vi "SolarPVLab.vi"(0 "SHDocVw.IWebBrowser2":refnum<k7>(container), 1 "location :":string, 2 "Go":bool) -> ()   [LabVIEW 2011]
doc: "To use this browser, you can type in a URL in the location field and then click on the Go button. You can also use the Back, Forward, Reload and Search buttons. This VI also has a runtime menu which is included in the library. When you run the VI, you will have File Menu and a History Menu. The file menu contains the same functionality that the buttons can do and the History menu contains a History of all the pages that you have visited in a given session.\n\nThe Invoke Node and Property Node functions are used to control the operation of the web browser. For more information on the Microsoft Web Browser Control, see Microsoft's web site (try http://support.microsoft.com/support/kb/articles/q165/2/12.asp)."
uses:
  2009 final/Solar Pv project Folder/SolarPVLab Folder/Voltage Array1.vi
panel:
  out "Current 150":dbl[](array[numeric])
  out "Voltage 150":dbl[](array[numeric])
  out "Current 130":dbl[](array[numeric])
  out "Voltage 130":dbl[](array[numeric])
  out "Current 100":dbl[](array[numeric])
  out "Voltage 100":dbl[](array[numeric])
  out "Current 60":dbl[](array[numeric])
  out "Voltage 60":dbl[](array[numeric])
  in  "stop":bool
  out "Video Feed":T1(plugin-control)
  in  "Tab Control":T2(tab)
  in  "Search":bool
  in  "Reload":bool
  in  "Back":bool
  in  "Forward":bool
  in  "Irradiation":T3(ring)
  in  "Resistance":T4(ring)
  in  "Angle of Incidence":T5(ring)
  out "Current Values Plotted":T6
  in  "Plot Current Values":T7
  in  "Plot Voltage Values":T8
  out "Voltage Values Plotted":T9
  in  "Tab Control 2":T10(tab)
  out "IV characeristics":cluster{"Y":dbl[], "Y":dbl[]}[](graph)
  out "Power vs Voltage":cluster{"Y":dbl[], "Y":dbl[]}[](graph)
  out "Current vs Incidence":cluster{"Y":dbl[], "Y":dbl[]}[](graph)
  out "Voltage vs Incidence":cluster{"Y":dbl[], "Y":dbl[]}[](graph)
  out "Irradiation Graph":cluster{dbl[], dbl[]}[](graph)
  out "Power varying with Irradiation Graph":cluster{dbl[], dbl[]}[](graph)
  out "Passing Array":string[](array[string])=["http://espn.go.com/", "http://www.natinst.com/"]
  # "WELCOME TO THE SOLAR PHOTOVOLTAIC LABORATORY\n\n\n\n\nTHIS SOLAR PHOTOVOLTAIC ILAB INVESTIGATES THE FOLLOWING \n                  CHARACTERISTICS OF A SOLAR PANEL:\n\n~CURRENT - VOLTAGE (IV) CHARACTERISITICS\n~VARIATION OF IV CHARACTERISITCS WITH IRRADIATION\n~VARIATION OF CURRENT AND VOLTAGE WITH ANGLE OF INCIDENCE\n\n\n\n\n\n\n© 2014 iLABS@MAK"
  # "* Select VI Info... from the Windows menu to find out how to use this example. *"
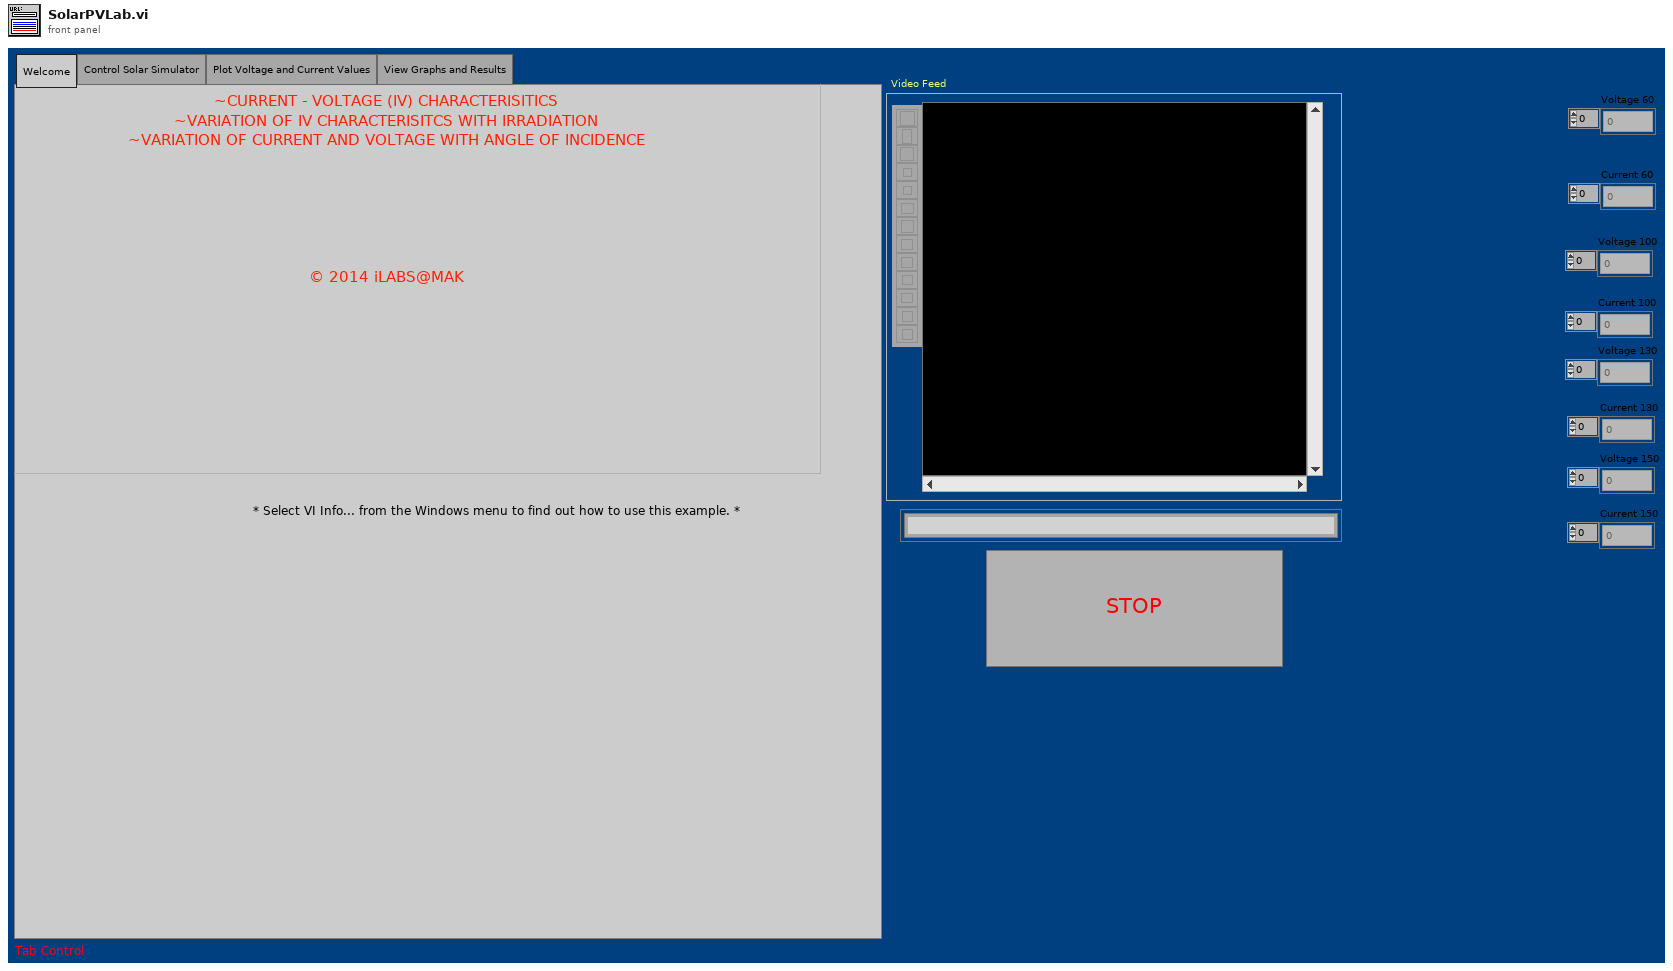
[diagram p1: front panel]
types:
  T1 = typedef "IMAQ Image.ctl" = refnum<image>
  T2 = enum32{"Welcome", "Control Solar Simulator", "Plot Voltage and Current Values", "View Graphs and Results"}
  T3 = enum16{"Choose Irradiation", "60", "100", "130", "150"}
  T4 = enum16{"Choose Resistance", "2.2 ohms", "4.7 ohms", "6.8 ohms", "8.2 ohms", "10 ohms", "12 ohms", "Shortciruit"}
  T5 = enum16{"0", "20", "40", "60", "80", "100", "120", "140", "160", "180"}
  T6 = cluster{"Short circuit\n current":dbl, "Value 1":dbl, "Value 2":dbl, "Value 3":dbl, "Value 4":dbl, "Value 5":dbl, "Value 6":dbl}
  T7 = cluster{"Plot Short \nCircuit current":bool, "Plot Value 2":bool, "Plot Value 3":bool, "Plot Value 4":bool, "Plot Value 5":bool, "Plot Value 6":bool, "Plot Value 7":bool}
  T8 = cluster{"Plot Value 1":bool, "Plot Value 2":bool, "Plot Value 3":bool, "Plot Value 4":bool, "Plot Value 5":bool, "Plot Value 6":bool, "Plot Open Circuit Voltage":bool}
  T9 = cluster{"Value 1":dbl, "Value 2":dbl, "Value 3":dbl, "Value 4":dbl, "Value 5":dbl, "Value 6":dbl, "Open circuit \n    Voltage":dbl}
  T10 = enum32{"IV Characteristics", "Power vs Voltage Graph", "Variation with Angle of Incidence", "IV-Variation with Irradiation", "Power-Irradiation Graph"}
  T11 = cluster{dynamicdata, dynamicdata, dynamicdata, dynamicdata, dynamicdata, dynamicdata, dynamicdata}
  T12 = cluster{"Voltage 150":dbl[], "Current 150":dbl[]}
  T13 = cluster{"Voltage 130":dbl[], "Current 130":dbl[]}
  T14 = cluster{"Voltage 100":dbl[], "Current 100":dbl[]}
  T15 = cluster{"Voltage 150":dbl[], "Current 150":dbl[]}[]
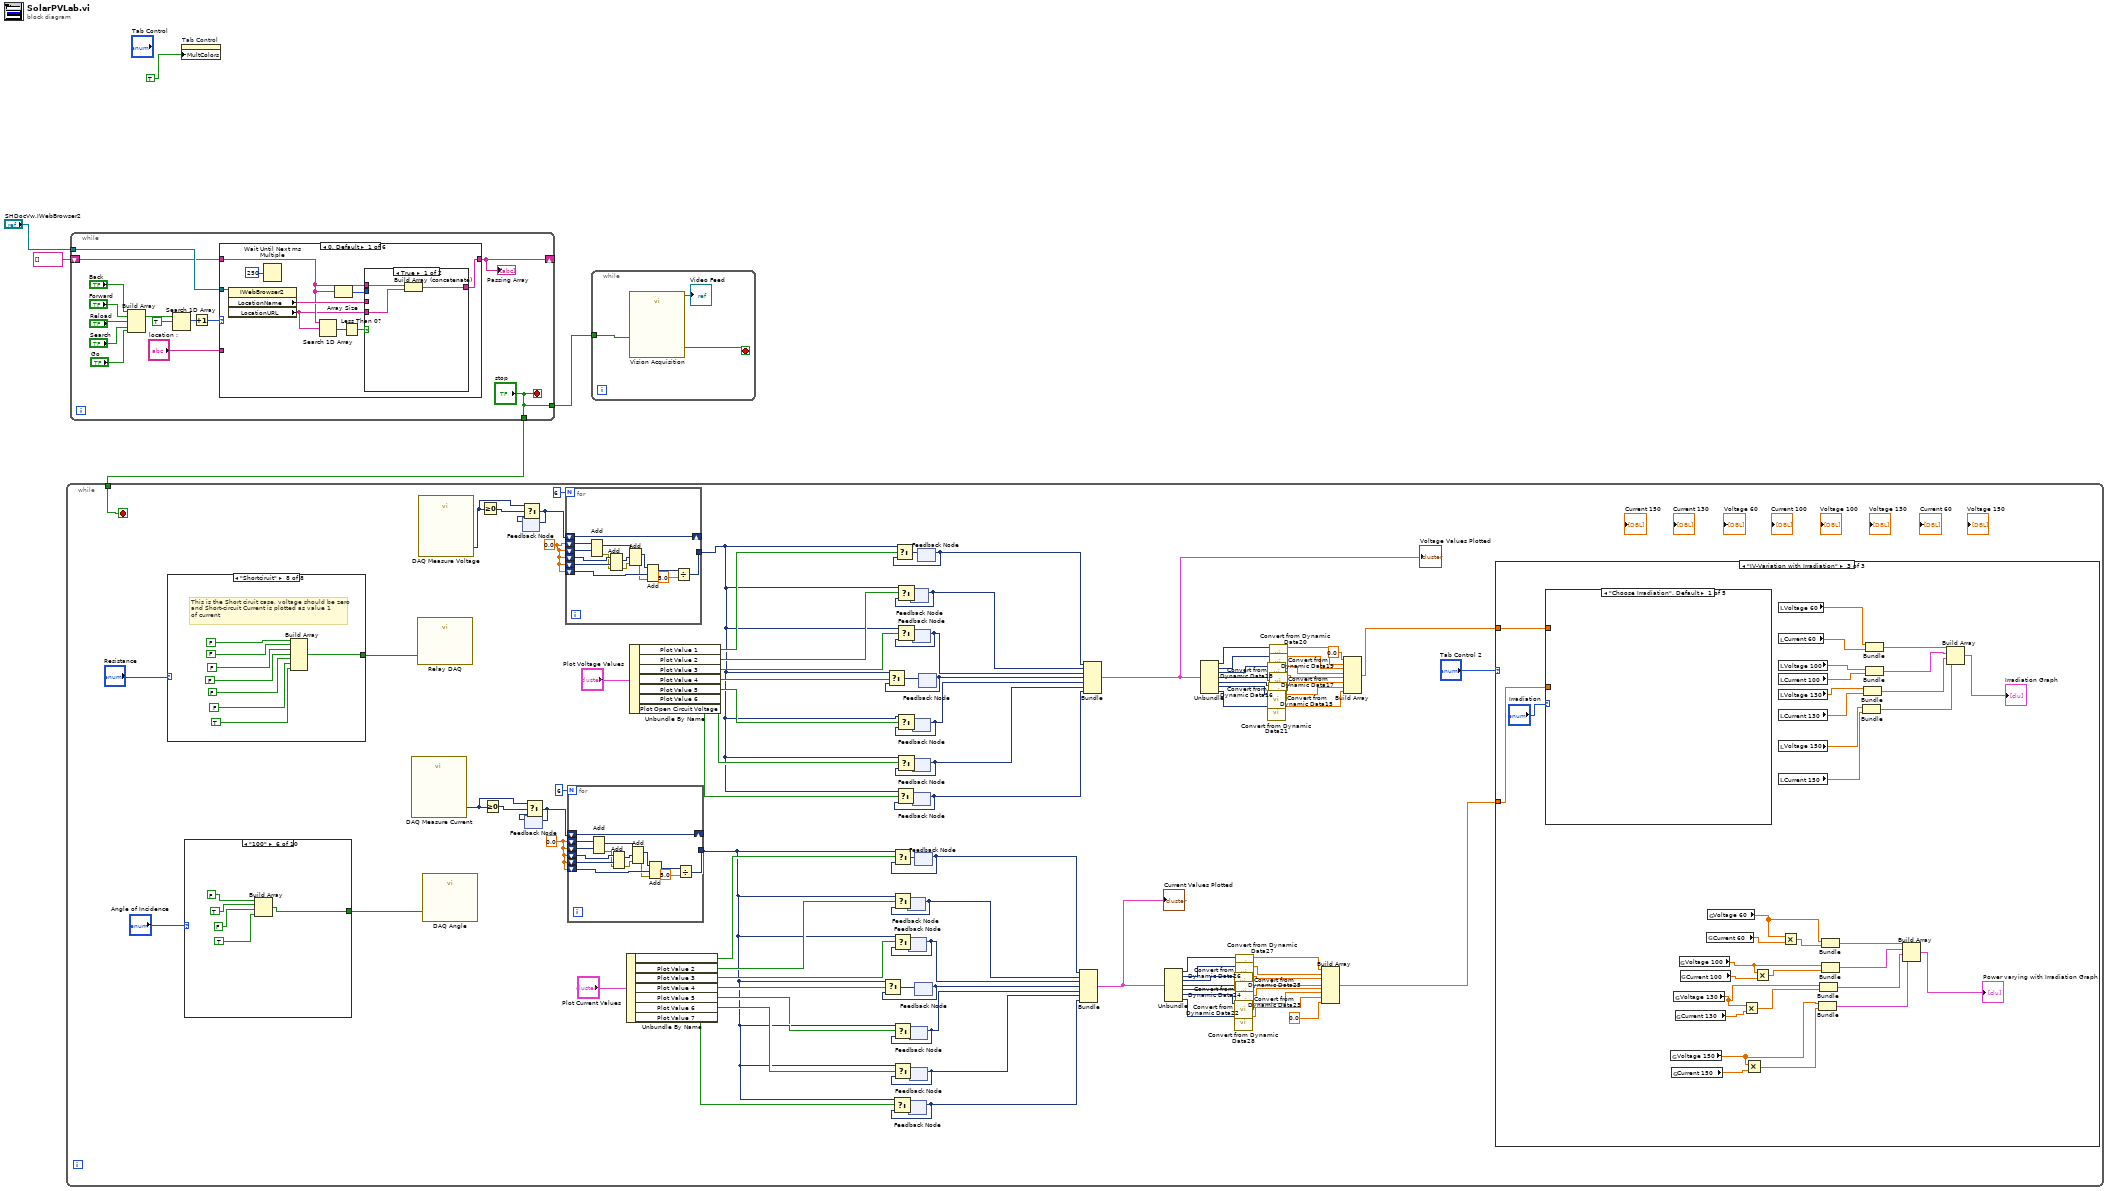
[diagram p0: block diagram]
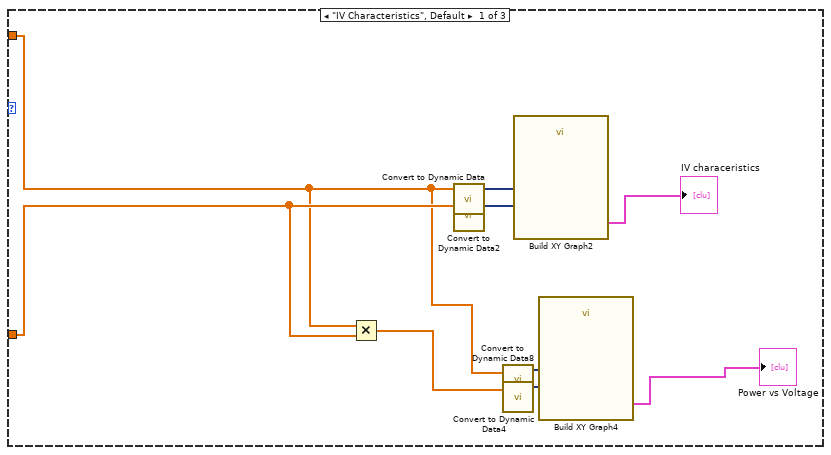
[diagram p2: hidden frame]
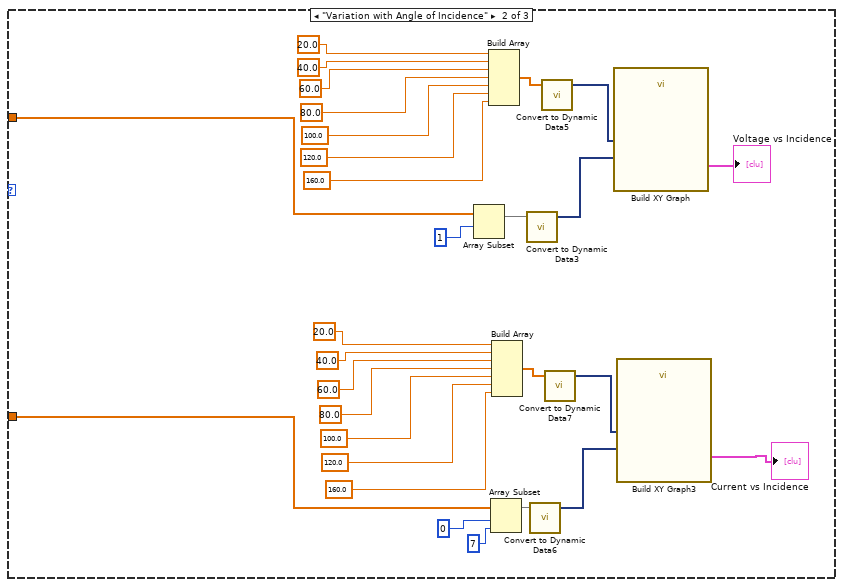
[diagram p3: hidden frame]
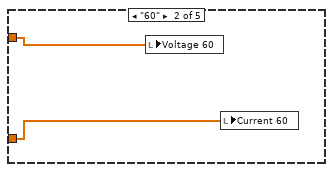
[diagram p4: hidden frame]
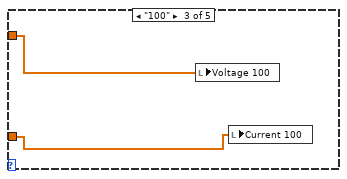
[diagram p5: hidden frame]
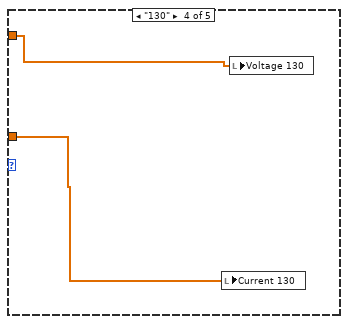
[diagram p6: hidden frame]
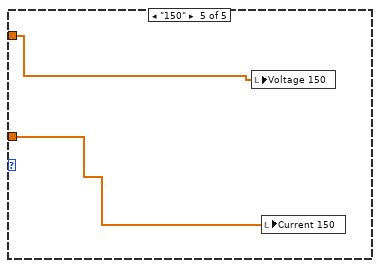
[diagram p7: hidden frame]
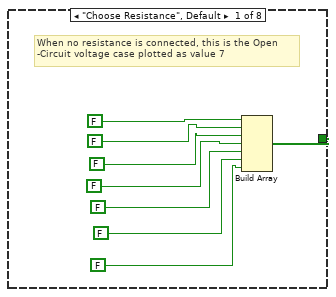
[diagram p8: hidden frame]
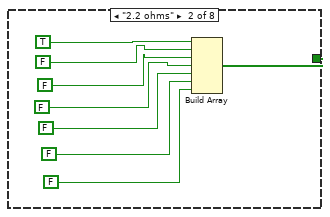
[diagram p9: hidden frame]
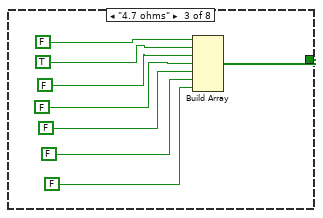
[diagram p10: hidden frame]
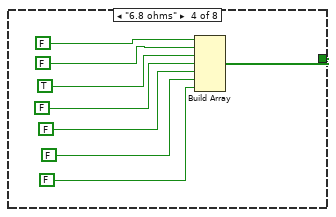
[diagram p11: hidden frame]
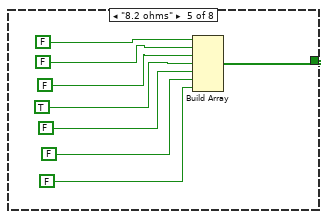
[diagram p12: hidden frame]
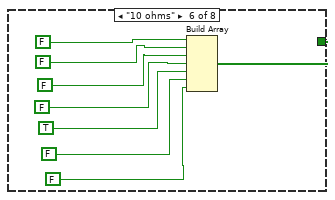
[diagram p13: hidden frame]
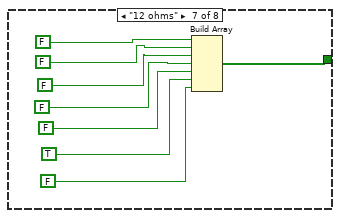
[diagram p14: hidden frame]
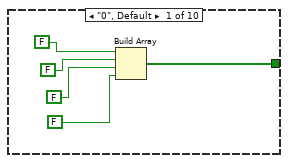
[diagram p15: hidden frame]
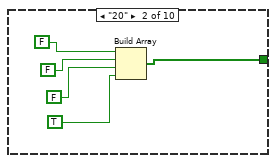
[diagram p16: hidden frame]
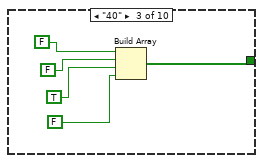
[diagram p17: hidden frame]
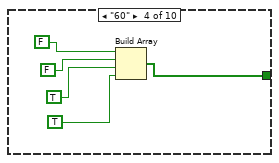
[diagram p18: hidden frame]
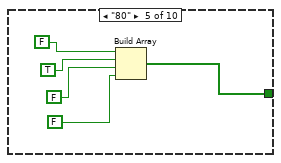
[diagram p19: hidden frame]
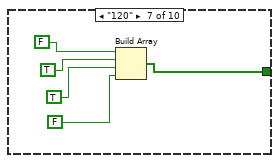
[diagram p20: hidden frame]
diagram:
  n1 = while {
    shift-left: string[] [] -> [w9]
    shift-right: [w8] -> _
    tunnel: "SHDocVw.IWebBrowser2" -> [w10]
    tunnel: ["stop"] -> w2
    tunnel: ["stop"] -> w1
    stop <- "stop" stop-if-true
    n2 = Build Array("Back", "Forward", "Reload", "Search", "Go") -> (w14:bool[])
    n3 = Search 1D Array(1D array=w14, element=TRUE) -> (index of element=w12:i32)  [unwired: 1 in]
    n4 = Increment(x=w12) -> (x+1=w11:i32)
    n5 = case shown="0, Default" w11 {
      tunnel: w10 -> [w20 w34 w36 w37 w39 w43]
      tunnel: "location :" -> [_ _ _ _ _ w42]
      tunnel: w9 -> [w24 w33 w35 w38 w40 w41]
      tunnel: [w23 w33 w35 w38 w40 w41] -> w8
      frame 0, Default {
        n6 = property class="IWebBrowser2"(reference=w20) -> ("LocationName"=w28:string, "LocationURL"=w21:string)  [unwired: 1 in, 2 out]
        n7 = Wait Until Next ms Multiple(millisecond multiple=u32 250) -> ()  [unwired: 1 out]
        n8 = Search 1D Array(1D array=w24, element=w21) -> (index of element=w27:i32)  [unwired: 1 in]
        n9 = Array Size(array=w24) -> (size(s)=w25:i32)
        n10 = Less Than 0?(x=w27) -> (x < 0?=w26:bool)
        n11 = case shown="True" w26 {
          tunnel: w28 -> [_ _]
          tunnel: w21 -> [w29 _]
          tunnel: w25 -> [_ _]
          tunnel: w24 -> [w31 w32]
          tunnel: [w30 w32] -> w23
          frame True {
            n12 = Build Array (concatenate)(w31, w29) -> (w30:string[])
          }
          frame False {
          }
        }
      }
      frame 1 {
        n13 = invoke class="IWebBrowser2" method="GoBack"(reference=w34) -> ()  [unwired: 2 in, 3 out]
      }
      frame 2 {
        n14 = invoke class="IWebBrowser2" method="GoForward"(reference=w36) -> ()  [unwired: 2 in, 3 out]
      }
      frame 3 {
        n15 = invoke class="IWebBrowser2" method="Refresh"(reference=w37) -> ()  [unwired: 2 in, 3 out]
      }
      frame 4 {
        n16 = invoke class="IWebBrowser2" method="GoSearch"(reference=w39) -> ()  [unwired: 2 in, 3 out]
      }
      frame 5 {
        n17 = invoke class="IWebBrowser2" method="Navigate"(reference=w43, "URL"=w42) -> ()  [unwired: 6 in, 8 out]
      }
    }
    "Passing Array" <- w8
  }
  n18 = while {
    tunnel: w2 -> [w44]
    stop <- w44 stop-if-true
    w45 = 0.0
    w46 = 0.0
    n19 = case shown="\"Shortciruit\"" "Resistance" {
      tunnel: [w252 w260 w268 w276 w284 w292 w300 w307] -> w139
      frame "Choose Resistance", Default {
        # "When no resistance is connected, this is the Open\n-Circuit voltage case plotted as value 7"
        n20 = Build Array(FALSE, FALSE, FALSE, FALSE, FALSE, FALSE, FALSE) -> (w252:bool[])
      }
      frame "2.2 ohms" {
        n21 = Build Array(TRUE, FALSE, FALSE, FALSE, FALSE, FALSE, FALSE) -> (w260:bool[])
      }
      frame "4.7 ohms" {
        n22 = Build Array(FALSE, TRUE, FALSE, FALSE, FALSE, FALSE, FALSE) -> (w268:bool[])
      }
      frame "6.8 ohms" {
        n23 = Build Array(FALSE, FALSE, TRUE, FALSE, FALSE, FALSE, FALSE) -> (w276:bool[])
      }
      frame "8.2 ohms" {
        n24 = Build Array(FALSE, FALSE, FALSE, TRUE, FALSE, FALSE, FALSE) -> (w284:bool[])
      }
      frame "10 ohms" {
        n25 = Build Array(FALSE, FALSE, FALSE, FALSE, TRUE, FALSE, FALSE) -> (w292:bool[])
      }
      frame "12 ohms" {
        n26 = Build Array(FALSE, FALSE, FALSE, FALSE, FALSE, TRUE, FALSE) -> (w300:bool[])
      }
      frame "Shortciruit" {
        # "This is the Short ciruit case, voltage should be zero \nand Short-circuit Current is plotted as value 1 \nof current"
        n27 = Build Array(FALSE, FALSE, FALSE, FALSE, FALSE, FALSE, TRUE) -> (w307:bool[])
      }
    }
    n28 = case shown="\"100\"" "Angle of Incidence" {
      tunnel: [w315 w320 w325 w330 w335 w340 w345 w350 w355 w360] -> w140
      frame "0", Default {
        n29 = Build Array(FALSE, FALSE, FALSE, FALSE) -> (w315:bool[])
      }
      frame "20" {
        n30 = Build Array(FALSE, FALSE, FALSE, TRUE) -> (w320:bool[])
      }
      frame "40" {
        n31 = Build Array(FALSE, FALSE, TRUE, FALSE) -> (w325:bool[])
      }
      frame "60" {
        n32 = Build Array(FALSE, FALSE, TRUE, TRUE) -> (w330:bool[])
      }
      frame "80" {
        n33 = Build Array(FALSE, TRUE, FALSE, FALSE) -> (w335:bool[])
      }
      frame "100" {
        n34 = Build Array(FALSE, TRUE, FALSE, TRUE) -> (w340:bool[])
      }
      frame "120" {
        n35 = Build Array(FALSE, TRUE, TRUE, FALSE) -> (w345:bool[])
      }
      frame "140" {
        n36 = Build Array(FALSE, TRUE, TRUE, TRUE) -> (w350:bool[])
      }
      frame "160" {
        n37 = Build Array(TRUE, FALSE, FALSE, FALSE) -> (w355:bool[])
      }
      frame "180" {
        n38 = Build Array(TRUE, FALSE, FALSE, TRUE) -> (w360:bool[])
      }
    }
    n39 = call "DAQ Measure Current"() -> ("data"=w57:dynamicdata)  [unwired: 17 in, 2 out]
    n40 = call "Relay DAQ"("data"=w139) -> ()  [unwired: 17 in, 2 out]
    n41 = call "DAQ Measure Voltage"() -> ("data"=w50:dynamicdata)  [unwired: 17 in, 2 out]
    n42 = call "DAQ Angle"("data"=w140) -> ()  [unwired: 17 in, 2 out]
    n43 = Greater Or Equal To 0?(x=w50) -> (x >= 0?=w53:dynamicdata)
    n44 = Greater Or Equal To 0?(x=w57) -> (x >= 0?=w58:dynamicdata)
    n45 = feedback #1() -> (w52:dynamicdata)  [unwired: 1 in]
    n46 = Select(t=w50, s=w53, f=w52) -> (s? t:f=w51:dynamicdata)
    n47 = feedback-in #1(w51) -> ()
    n48 = feedback #2() -> (w56:dynamicdata)  [unwired: 1 in]
    n49 = Select(t=w57, s=w58, f=w56) -> (s? t:f=w55:dynamicdata)
    n50 = feedback-in #2(w55) -> ()
    n51 = for {
      N: 6 -> [_]
      shift-right: [w156] -> _
      shift-left: w51 -> [w156]
      shift-left: w45 -> [w155]
      shift-left: w45 -> [w154]
      shift-left: w45 -> [w153]
      shift-left: w45 -> [w152]
      shift-left: w45 -> [w148]
      tunnel: [w145] -> w49
      n52 = Add(1:w154, 2:w155) -> (0:w151:dynamicdata, 3:w144:errorcluster)  [unwired: 1 in]
      n53 = Add(1:w152, 2:w153, 4:w144) -> (0:w150:dynamicdata, 3:w143:errorcluster)
      n54 = Add(1:w150, 2:w151, 4:w143) -> (0:w149:dynamicdata, 3:w142:errorcluster)
      n55 = Add(1:w148, 2:w149, 4:w142) -> (0:w147:dynamicdata)  [unwired: 1 out]
      n56 = Divide(x=w147, y=5.0) -> (x/y=w145:dynamicdata)
    }
    n57 = for {
      N: 6 -> [_]
      shift-right: [w171] -> _
      shift-left: w55 -> [w171]
      shift-left: w46 -> [w170]
      shift-left: w46 -> [w169]
      shift-left: w46 -> [w168]
      shift-left: w46 -> [w167]
      shift-left: w46 -> [w163]
      tunnel: [w160] -> w54
      n58 = Add(1:w169, 2:w170) -> (0:w166:dynamicdata, 3:w159:errorcluster)  [unwired: 1 in]
      n59 = Add(1:w167, 2:w168, 4:w159) -> (0:w165:dynamicdata, 3:w158:errorcluster)
      n60 = Add(1:w165, 2:w166, 4:w158) -> (0:w164:dynamicdata, 3:w157:errorcluster)
      n61 = Add(1:w163, 2:w164, 4:w157) -> (0:w162:dynamicdata)  [unwired: 1 out]
      n62 = Divide(x=w162, y=5.0) -> (x/y=w160:dynamicdata)
    }
    n63 = Unbundle By Name("Plot Current Values") -> ("Plot Short \nCircuit current"=w103:bool, "Plot Value 2"=w102:bool, "Plot Value 3"=w101:bool, "Plot Value 4"=w100:bool, "Plot Value 5"=w99:bool, "Plot Value 6"=w59:bool, "Plot Value 7"=w79:bool)
    n64 = Unbundle By Name("Plot Voltage Values") -> ("Plot Value 1"=w68:bool, "Plot Value 2"=w67:bool, "Plot Value 3"=w66:bool, "Plot Value 4"=w65:bool, "Plot Value 5"=w64:bool, "Plot Value 6"=w63:bool, "Plot Open Circuit Voltage"=w62:bool)
    n65 = feedback #3() -> (w98:dynamicdata)  [unwired: 1 in]
    n66 = Select(t=w54, s=w102, f=w98) -> (s? t:f=w108:dynamicdata)
    n67 = feedback-in #3(w108) -> ()
    n68 = feedback #4() -> (w97:dynamicdata)  [unwired: 1 in]
    n69 = Select(t=w54, s=w101, f=w97) -> (s? t:f=w107:dynamicdata)
    n70 = feedback-in #4(w107) -> ()
    n71 = feedback #5() -> (w78:dynamicdata)  [unwired: 1 in]
    n72 = Select(t=w54, s=w79, f=w78) -> (s? t:f=w80:dynamicdata)
    n73 = feedback-in #5(w80) -> ()
    n74 = feedback #6() -> (w95:dynamicdata)  [unwired: 1 in]
    n75 = Select(t=w54, s=w99, f=w95) -> (s? t:f=w105:dynamicdata)
    n76 = feedback-in #6(w105) -> ()
    n77 = feedback #7() -> (w94:dynamicdata)  [unwired: 1 in]
    n78 = Select(t=w54, s=w59, f=w94) -> (s? t:f=w104:dynamicdata)
    n79 = feedback-in #7(w104) -> ()
    n80 = feedback #8() -> (w129:dynamicdata)  [unwired: 1 in]
    n81 = Select(t=w49, s=w67, f=w129) -> (s? t:f=w134:dynamicdata)
    n82 = feedback-in #8(w134) -> ()
    n83 = feedback #9() -> (w128:dynamicdata)  [unwired: 1 in]
    n84 = Select(t=w49, s=w66, f=w128) -> (s? t:f=w133:dynamicdata)
    n85 = feedback-in #9(w133) -> ()
    n86 = feedback #10() -> (w74:dynamicdata)  [unwired: 1 in]
    n87 = Select(t=w49, s=w62, f=w74) -> (s? t:f=w111:dynamicdata)
    n88 = feedback-in #10(w111) -> ()
    n89 = feedback #11() -> (w126:dynamicdata)  [unwired: 1 in]
    n90 = Select(t=w49, s=w64, f=w126) -> (s? t:f=w131:dynamicdata)
    n91 = feedback-in #11(w131) -> ()
    n92 = feedback #12() -> (w125:dynamicdata)  [unwired: 1 in]
    n93 = Select(t=w49, s=w63, f=w125) -> (s? t:f=w130:dynamicdata)
    n94 = feedback-in #12(w130) -> ()
    n95 = feedback #13() -> (w93:dynamicdata)  [unwired: 1 in]
    n96 = Select(t=w54, s=w103, f=w93) -> (s? t:f=w109:dynamicdata)
    n97 = feedback-in #13(w109) -> ()
    n98 = feedback #14() -> (w96:dynamicdata)  [unwired: 1 in]
    n99 = Select(t=w54, s=w100, f=w96) -> (s? t:f=w106:dynamicdata)
    n100 = feedback-in #14(w106) -> ()
    n101 = feedback #15() -> (w124:dynamicdata)  [unwired: 1 in]
    n102 = Select(t=w49, s=w68, f=w124) -> (s? t:f=w135:dynamicdata)
    n103 = feedback-in #15(w135) -> ()
    n104 = feedback #16() -> (w127:dynamicdata)  [unwired: 1 in]
    n105 = Select(t=w49, s=w65, f=w127) -> (s? t:f=w132:dynamicdata)
    n106 = feedback-in #16(w132) -> ()
    n107 = Bundle(w93, w98, w97, w96, w95, w94, w78) -> (w60:T11)  [unwired: 1 in]
    "Current Values Plotted" <- w60
    n108 = Bundle(w124, w129, w128, w127, w126, w125, w74) -> (w61:T11)  [unwired: 1 in]
    "Voltage Values Plotted" <- w61
    n109 = Unbundle(w60) -> (w92:dynamicdata, w91:dynamicdata, w90:dynamicdata, w89:dynamicdata, w88:dynamicdata, w87:dynamicdata, w77:dynamicdata)
    n110 = Unbundle(w61) -> (w123:dynamicdata, w122:dynamicdata, w121:dynamicdata, w120:dynamicdata, w119:dynamicdata, w118:dynamicdata, w73:dynamicdata)
    n111 = call "Convert from Dynamic Data22"("Dynamic Data Type"=w87) -> ("Scalar"=w81:dbl)  [unwired: 3 in]
    n112 = call "Convert from Dynamic Data28"("Dynamic Data Type"=w77) -> ("Scalar"=w76:dbl)  [unwired: 3 in]
    n113 = call "Convert from Dynamic Data25"("Dynamic Data Type"=w90) -> ("Scalar"=w84:dbl)  [unwired: 3 in]
    n114 = call "Convert from Dynamic Data23"("Dynamic Data Type"=w88) -> ("Scalar"=w82:dbl)  [unwired: 3 in]
    n115 = call "Convert from Dynamic Data27"("Dynamic Data Type"=w92) -> ("Scalar"=w86:dbl)  [unwired: 3 in]
    n116 = call "Convert from Dynamic Data26"("Dynamic Data Type"=w91) -> ("Scalar"=w85:dbl)  [unwired: 3 in]
    n117 = call "Convert from Dynamic Data24"("Dynamic Data Type"=w89) -> ("Scalar"=w83:dbl)  [unwired: 3 in]
    n118 = call "Convert from Dynamic Data15"("Dynamic Data Type"=w118) -> ("Scalar"=w112:dbl)  [unwired: 3 in]
    n119 = call "Convert from Dynamic Data21"("Dynamic Data Type"=w73) -> ("Scalar"=w110:dbl)  [unwired: 3 in]
    n120 = call "Convert from Dynamic Data18"("Dynamic Data Type"=w121) -> ("Scalar"=w115:dbl)  [unwired: 3 in]
    n121 = call "Convert from Dynamic Data16"("Dynamic Data Type"=w119) -> ("Scalar"=w113:dbl)  [unwired: 3 in]
    n122 = call "Convert from Dynamic Data20"("Dynamic Data Type"=w123) -> ("Scalar"=w117:dbl)  [unwired: 3 in]
    n123 = call "Convert from Dynamic Data19"("Dynamic Data Type"=w122) -> ("Scalar"=w116:dbl)  [unwired: 3 in]
    n124 = call "Convert from Dynamic Data17"("Dynamic Data Type"=w120) -> ("Scalar"=w114:dbl)  [unwired: 3 in]
    n125 = Build Array(w86, w85, w84, w83, w82, w81, w76, 0.0 ("element")) -> (w69:dbl[])
    n126 = Build Array(0.0 ("element"), w117, w116, w115, w114, w113, w112, w110) -> (w70:dbl[])
    n127 = case shown="\"IV-Variation with Irradiation\"" "Tab Control 2" {
      tunnel: w70 -> [w176 w198 w241]
      tunnel: w69 -> [w179 w183 w240]
      frame "IV Characteristics", Default {
        n128 = Multiply(x=w176, y=w179) -> (x*y=w178:dbl[])
        n129 = call "Convert to Dynamic Data"("Array"=w176) -> ("Dynamic Data Type"=w172:dynamicdata)  [unwired: 3 in]
        n130 = call "Convert to Dynamic Data2"("Array"=w179) -> ("Dynamic Data Type"=w180:dynamicdata)  [unwired: 3 in]
        n131 = call "Convert to Dynamic Data8"("Array"=w176) -> ("Dynamic Data Type"=w175:dynamicdata)  [unwired: 3 in]
        n132 = call "Convert to Dynamic Data4"("Array"=w178) -> ("Dynamic Data Type"=w177:dynamicdata)  [unwired: 3 in]
        n133 = call "Build XY Graph2"("Y Input"=w180, "X Input"=w172) -> ("XY Graph"=→"IV characeristics":cluster{"Y":dbl[], "Y":dbl[]}[])  [unwired: 3 in, 6 out]
        n134 = call "Build XY Graph4"("Y Input"=w177, "X Input"=w175) -> ("XY Graph"=→"Power vs Voltage":cluster{"Y":dbl[], "Y":dbl[]}[])  [unwired: 3 in, 6 out]
      }
      frame "Variation with Angle of Incidence" {
        n135 = Array Subset(array=w198, index=1) -> (w196:dbl[])  [unwired: 1 in]
        n136 = Build Array(20.0 ("element"), 40.0 ("element"), 60.0 ("element"), 80.0 ("element"), 100.0 ("element"), 120.0 ("element"), 160.0 ("element")) -> (w207:dbl[])
        n137 = Array Subset(array=w183, index=0, length=7) -> (w184:dbl[])
        n138 = Build Array(20.0 ("element"), 40.0 ("element"), 60.0 ("element"), 80.0 ("element"), 100.0 ("element"), 120.0 ("element"), 160.0 ("element")) -> (w194:dbl[])
        n139 = call "Convert to Dynamic Data3"("Array"=w196) -> ("Dynamic Data Type"=w208:dynamicdata)  [unwired: 3 in]
        n140 = call "Convert to Dynamic Data6"("Array"=w184) -> ("Dynamic Data Type"=w195:dynamicdata)  [unwired: 3 in]
        n141 = call "Convert to Dynamic Data5"("Array"=w207) -> ("Dynamic Data Type"=w206:dynamicdata)  [unwired: 3 in]
        n142 = call "Convert to Dynamic Data7"("Array"=w194) -> ("Dynamic Data Type"=w193:dynamicdata)  [unwired: 3 in]
        n143 = call "Build XY Graph"("Y Input"=w208, "X Input"=w206) -> ("XY Graph"=→"Voltage vs Incidence":cluster{"Y":dbl[], "Y":dbl[]}[])  [unwired: 3 in, 6 out]
        n144 = call "Build XY Graph3"("Y Input"=w195, "X Input"=w193) -> ("XY Graph"=→"Current vs Incidence":cluster{"Y":dbl[], "Y":dbl[]}[])  [unwired: 3 in, 6 out]
      }
      frame "IV-Variation with Irradiation" {
        n145 = case shown="\"Choose Irradiation\", Default" "Irradiation" {
          tunnel: w241 -> [_ w244 w246 w248 w250]
          tunnel: w240 -> [_ w243 w245 w247 w249]
          frame "Choose Irradiation", Default {
          }
          frame "60" {
            n146 = local write "Voltage 60"(w244) -> ()
            n147 = local write "Current 60"(w243) -> ()
          }
          frame "100" {
            n148 = local write "Voltage 100"(w246) -> ()
            n149 = local write "Current 100"(w245) -> ()
          }
          frame "130" {
            n150 = local write "Current 130"(w247) -> ()
            n151 = local write "Voltage 130"(w248) -> ()
          }
          frame "150" {
            n152 = local write "Voltage 150"(w250) -> ()
            n153 = local write "Current 150"(w249) -> ()
          }
        }
        n154 = global read "Voltage Array1.vi" "Voltage 150"() -> (w219:dbl[])
        n155 = global read "Voltage Array1.vi" "Current 150"() -> (w221:dbl[])
        n156 = global read "Voltage Array1.vi" "Voltage 130"() -> (w222:dbl[])
        n157 = global read "Voltage Array1.vi" "Current 130"() -> (w224:dbl[])
        n158 = global read "Voltage Array1.vi" "Voltage 100"() -> (w225:dbl[])
        n159 = global read "Voltage Array1.vi" "Current 100"() -> (w227:dbl[])
        n160 = global read "Voltage Array1.vi" "Current 60"() -> (w230:dbl[])
        n161 = global read "Voltage Array1.vi" "Voltage 60"() -> (w228:dbl[])
        n162 = Multiply(x=w222, y=w224) -> (x*y=w223:dbl[])
        n163 = Multiply(x=w219, y=w221) -> (x*y=w220:dbl[])
        n164 = Multiply(x=w225, y=w227) -> (x*y=w226:dbl[])
        n165 = local read "Voltage 60"() -> (w217:dbl[])
        n166 = local read "Current 60"() -> (w216:dbl[])
        n167 = local read "Voltage 100"() -> (w215:dbl[])
        n168 = local read "Current 100"() -> (w214:dbl[])
        n169 = local read "Voltage 130"() -> (w213:dbl[])
        n170 = local read "Current 130"() -> (w212:dbl[])
        n171 = local read "Voltage 150"() -> (w211:dbl[])
        n172 = local read "Current 150"() -> (w210:dbl[])
        n173 = Multiply(x=w228, y=w230) -> (x*y=w229:dbl[])
        n174 = Bundle("Voltage 150"=w219, w220) -> (w233:cluster{"Voltage 150":dbl[], dbl[]})  [unwired: 1 in]
        n175 = Bundle("Voltage 130"=w222, w223) -> (w234:cluster{"Voltage 130":dbl[], dbl[]})  [unwired: 1 in]
        n176 = Bundle("Voltage 60"=w228, w229) -> (w231:cluster{"Voltage 60":dbl[], dbl[]})  [unwired: 1 in]
        n177 = Bundle("Voltage 100"=w225, w226) -> (w232:cluster{"Voltage 100":dbl[], dbl[]})  [unwired: 1 in]
        n178 = Bundle("Voltage 150"=w211, "Current 150"=w210) -> (w237:T12)  [unwired: 1 in]
        n179 = Bundle("Voltage 130"=w213, "Current 130"=w212) -> (w238:T13)  [unwired: 1 in]
        n180 = Bundle("Voltage 60"=w217, "Current 60"=w216) -> (w235:cluster{"Voltage 60":dbl[], "Current 60":dbl[]})  [unwired: 1 in]
        n181 = Bundle("Voltage 100"=w215, "Current 100"=w214) -> (w236:T14)  [unwired: 1 in]
        n182 = Build Array(w231, w232, w234, w233) -> (→"Power varying with Irradiation Graph":cluster{"Voltage 150":dbl[], dbl[]}[])
        n183 = Build Array(w235, w236, w238, w237) -> (→"Irradiation Graph":T15)
      }
    }
  }
  n184 = property on="Tab Control" class="TabCtl (strict)"("MultColors"=TRUE) -> ()  [unwired: 2 in, 2 out]
  n185 = while {
    tunnel: w1 -> [w365]
    stop <- w366 stop-if-true
    n186 = call "Vision Acquisition"("Stop (F)"=w365) -> ("Image Out"=→"Video Feed":T1, "Stopped"=w366:bool)  [unwired: 24 in, 1 out]
  }
